vi "CC Script Unwind.vi"(8 "error in (no error)":errorcluster, 9 "Script Path":path, 10 "Indent":i32, 11 "Script":T3) -> (0 "error out":errorcluster, 2 "Indent":i32[](array[numeric]), 3 "Unwound Script":T1[](array[typedef]))   [LabVIEW 2024]
uses:
  typedefs/CC cluster Script.ctl
  typedefs/CC Script Step.ctl
  typedefs/CC enum Script Action.ctl
panel:
  out "Callers":string[](array[string])
  in  "Caller":string
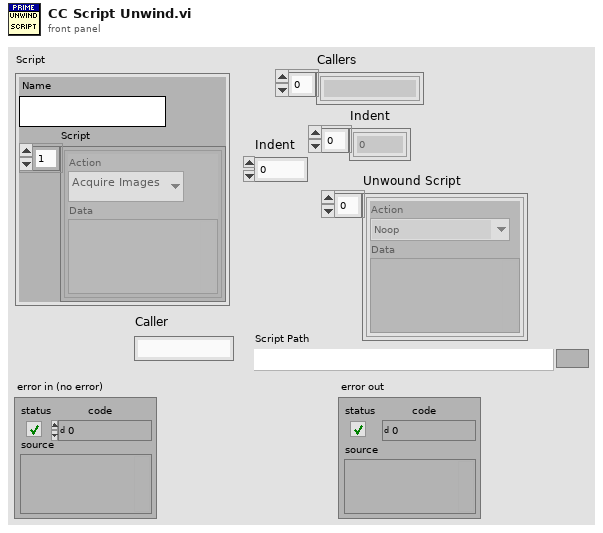
[diagram p1: front panel]
types:
  T1 = typedef "CC Script Step.ctl" = cluster{"Action":T2, "Data":variant}
  T2 = typedef "CC enum Script Action.ctl" = enum16{"Noop", "Define Object", "Define Exposure", "Define Dithering", "Acquire Images", "Set Filter Wheel", "Telescope Home", "Telescope Move", "Telescope RA DEC", "Focus Move Relative", "Focus Move Absolute", "Focus Set Home", "Macro", "Pause", "Ask User", "Define Random Dither", "CmdLine", "Outlet"}
  T3 = typedef "CC cluster Script.ctl" = cluster{"Name":string, "Script":T1[]}
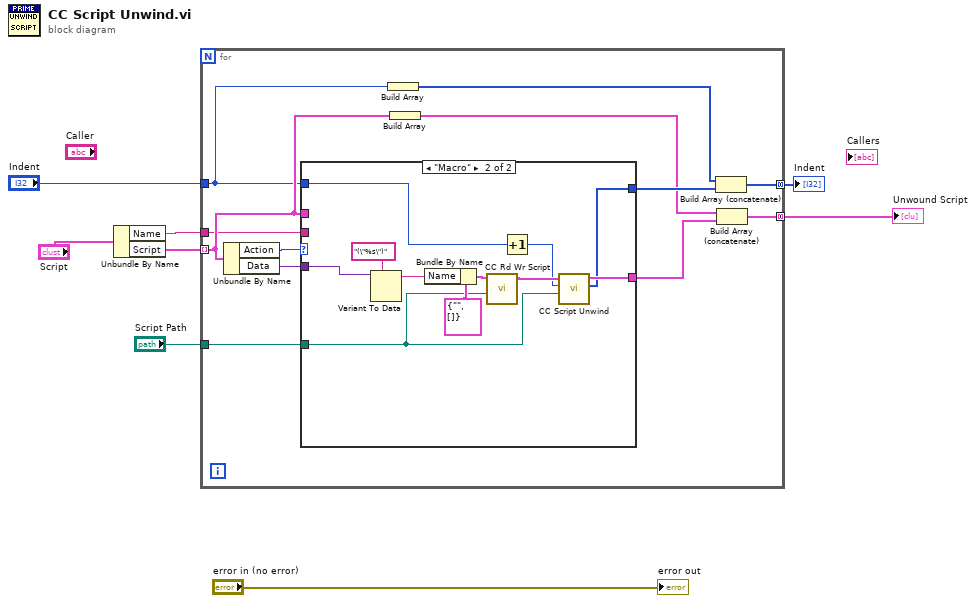
[diagram p0: block diagram]
diagram:
  n1 = Unbundle By Name("Script") -> ("Name"=w4:string, "Script"=w6:T1[])
  n2 = for {
    tunnel: w6 -> [w16] mode=indexing
    tunnel: [w18] -> w5 mode=concatenating
    tunnel: "Indent" -> [w15]
    tunnel: [w14] -> w2 mode=concatenating
    tunnel: w4 -> [w13]
    tunnel: "Script Path" -> [w9]
    n3 = Unbundle By Name(w16) -> ("Action"=w19:T2, "Data"=w20:variant)
    n4 = case shown="\"Macro\"" w19 {
      tunnel: w20 -> [_ w30]
      tunnel: [_ w25] -> w17
      tunnel: w16 -> [_ _]
      tunnel: w15 -> [_ w22]
      tunnel: w13 -> [_ _]
      tunnel: [_ w23] -> w12
      tunnel: w9 -> [_ w21]
      frame "Noop", Default {
      }
      frame "Macro" {
        n5 = Variant To Data(type="(\"%s\")" ("format string"), Variant=w30) -> (data=w26:string)  [unwired: 1 in, 1 out]
        n6 = Bundle By Name(cluster=T3 {"Name"="", "Script"=[]} ("Script"), "Name"=w26) -> (w28:T3)
        n7 = call "CC Rd Wr Script.vi"("Script Path"=w21, "Script"=w28) -> ("Script"=w27:T3)  [unwired: 4 in, 5 out]
        n8 = Increment(x=w22) -> (x+1=w24:i32)
        n9 = call "CC Script Unwind.vi"("Script Path"=w21, "Indent"=w24, "Script"=w27) -> ("Indent"=w23:i32[], "Unwound Script"=w25:T1[])  [unwired: 6 in, 1 out]
      }
    }
    n10 = Build Array(w15) -> (w11:i32[])
    n11 = Build Array(w16) -> (w10:T1[])
    n12 = Build Array (concatenate)(w11, w12) -> (w14:i32[])
    n13 = Build Array (concatenate)(w10, w17) -> (w18:T1[])
  }
  "Unwound Script" <- w5
  "Indent" <- w2
  "error out" <- "error in (no error)"
